vi "Go_to_Init.vi"(8 "error in (no error)":errorcluster, 11 "Init_cls in":refnum<class "Init_cls.lvclass">) -> (0 "error out":errorcluster, 3 "State out":refnum<class "State Actor.lvclass">)   [LabVIEW 2025, in "Demo_States.lvlib" / "Init_cls.lvclass"]
uses:
  Init_cls.lvclass
  <vilib>/ni/Actors/State Actor/State Actor/State Actor.lvclass
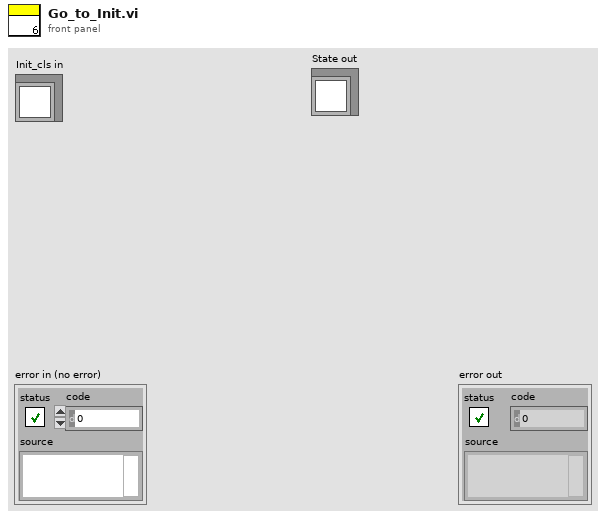
[diagram p1: front panel]
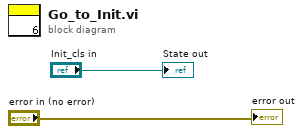
[diagram p0: block diagram]
diagram:
  "error out" <- "error in (no error)"
  "State out" <- "Init_cls in"
